vi "Configuration - Load.vi"(8 "error in (no error)":errorcluster, 11 "Configuration Data":T1) -> (0 "error out":errorcluster, 3 "Configuration Data":T1)   [LabVIEW 2017]
doc: "Reads configuration data from the external XML file"
uses:
  Controls/Configuration Data.ctl
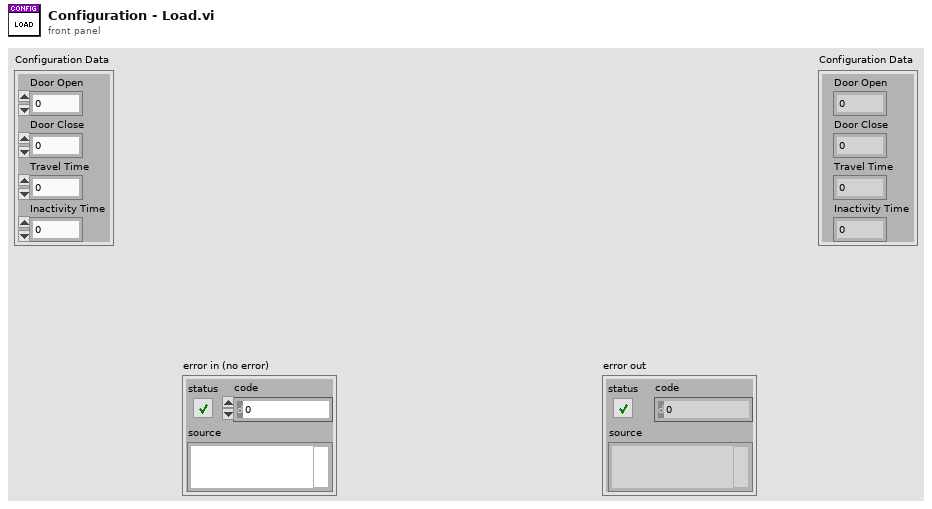
[diagram p1: front panel]
types:
  T1 = typedef "Configuration Data.ctl" = cluster{"Door Open":dbl, "Door Close":dbl, "Travel Time":dbl, "Inactivity Time":dbl}
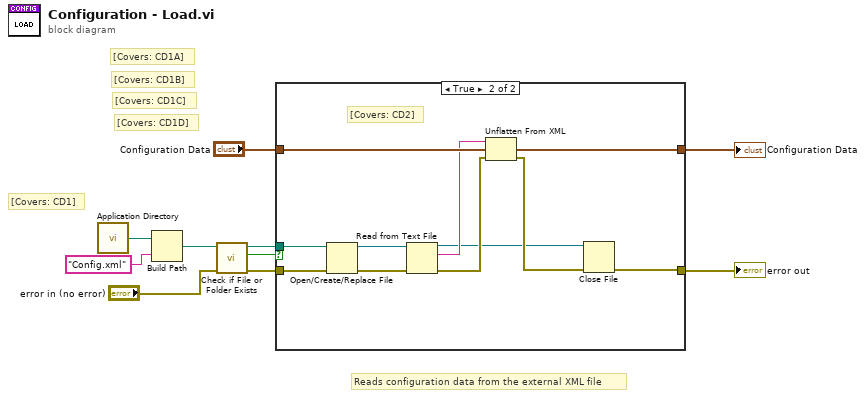
[diagram p0: block diagram]
diagram:
  # "[Covers: CD1D]"
  # "[Covers: CD1C]"
  # "[Covers: CD1B]"
  # "[Covers: CD1A]"
  # "[Covers: CD1]"
  # "Reads configuration data from the external XML file"
  n1 = call <vilib>:"Application Directory.vi"() -> ("Application Directory"=w10:path)
  n2 = Build Path(base path=w10, name or relative path="Config.xml") -> (appended path=w8:path)
  n3 = call <vilib>:"Check if File or Folder Exists.vi"("error in (no error)"="error in (no error)", "path"=w8) -> ("error out"=w4:errorcluster, "file or folder exists?"=w6:bool, "dup path"=w5:path)  [unwired: 7 in]
  n4 = case shown="True" w6 {
    tunnel: w5 -> [_ w22]
    tunnel: w4 -> [w12 w23]
    tunnel: [w12 w14] -> w3
    tunnel: "Configuration Data" -> [w11 w19]
    tunnel: [w11 w13] -> w1
    frame False {
      # "Create new config file and write default changes"
      # "[Covers: CD3]"
    }
    frame True {
      # "[Covers: CD2]"
      n5 = Open/Create/Replace File(file path (use dialog)=w22, error in=w23) -> (refnum out=w20:refnum<file>, error out=w21:errorcluster)  [unwired: 4 in, 1 out]
      n6 = Read from Text File(file (use dialog)=w20, error in=w21) -> (refnum out=w15:refnum<file>, text=w18:string, error out=w17:errorcluster)  [unwired: 2 in, 1 out]
      n7 = Unflatten From XML(xml string=w18, type=w19, error in (no error)=w17) -> (value=w13:T1, error out=w16:errorcluster)
      n8 = Close File(refnum=w15, error in=w16) -> (error out=w14:errorcluster)  [unwired: 1 out]
    }
  }
  "Configuration Data" <- w1
  "error out" <- w3
